vi "Configure Capture Analyzer Measurement.vi"(7 "Step (1)":i32=1, 8 "error in (no error)":errorcluster, 9 "Segment (1)":i32=1, 10 "Instance (1)":i32=1, 11 "VISA resource name":refnum<visa-resource-name>) -> (0 "error out":errorcluster, 3 "VISA resource name out":refnum<visa-resource-name>)   [LabVIEW 2020, in "Rohde&Schwarz CMXP GPRF.lvlib"]
doc: "Configures the capture analyzer measurement.\n\nAttributes:\nRSCMXPGPRF_ATTR_CAPTURE_ANALYZER_MEASUREMENT_SEGMENT\nRSCMXPGPRF_ATTR_CAPTURE_ANALYZER_MEASUREMENT_STEP\n\nRemote-control commands:\nCONFigure:GPRF:MEAS<i>:CANalyzer:SEGMent\nCONFigure:GPRF:MEAS<i>:CANalyzer:STEP"
uses:
  <instrlib>/Rohde&Schwarz CMXP GPRF/Rohde&Schwarz CMXP GPRF.lvlib
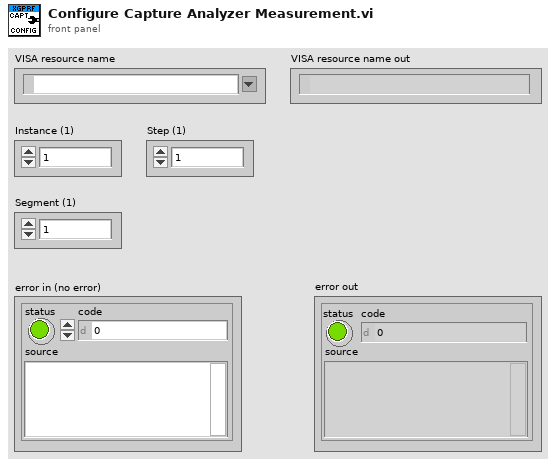
[diagram p1: front panel]
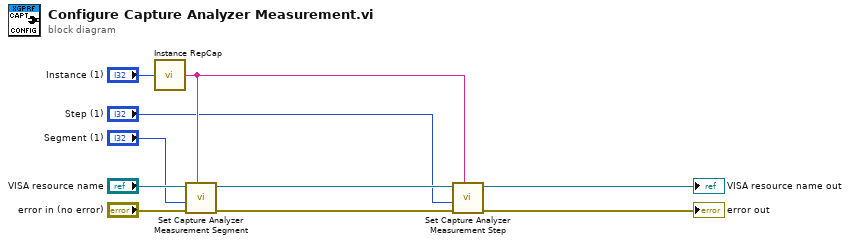
[diagram p0: block diagram]
diagram:
  n1 = call <instrlib>:"Instance RepCap.vi"("Instance in"="Instance (1)") -> ("Instance out"=w3:string)
  n2 = call "Set Capture Analyzer Measurement Segment"("Repeated Capabilities"=w3, "error in (no error)"="error in (no error)", "Capture Analyzer Measurement Segment (0)"="Segment (1)", "instrument handle"="VISA resource name") -> ("error out"=w5:errorcluster, "instrument handle out"=w6:refnum<visa-resource-name>)  [unwired: 6 in]
  n3 = call "Set Capture Analyzer Measurement Step"("Repeated Capabilities"=w3, "error in (no error)"=w5, "Capture Analyzer Measurement Step (0)"="Step (1)", "instrument handle"=w6) -> ("error out"=→"error out":errorcluster, "instrument handle out"=→"VISA resource name out":refnum<visa-resource-name>)  [unwired: 6 in]
